vi "Meadowlark USB IO Example v1.1.VI"(0 "Set Voltage":dbl min=0.0 max=10.0 step=0.001 format="%.3f", 5 "error in (no error)":errorcluster) -> (14 "Readout \nVoltages":dbl[](array[numeric]) format="%.3f", 19 "error out":errorcluster)   [LabVIEW 2010]
doc: "This example selects channels and sets and reads voltages on a Meadowlark Optics D3040 Four-Cell controller. This VI can be opened and examined using LabVIEW (6.1 or newer) as a starting point for a user's custom development of a D3040 interface. Please note that the Sub-VI's used in this program require the file \"usbdrvd.dll\".\n\n(c) 2002-2003 Meadowlark Optics, Inc. All rights reserved."
panel:
  out "FW Version":dbl=2.0 min=0.0 max=10.0 step=0.001 format="%.2f"
  out "Update \nChannel":bool[](array[boolean])
  out "Located USB Devices":bool[](array[boolean])=[TRUE]
  in  "stop":bool
  in  "USB Device Number":i32=1 min=1 max=1
  in  "Channel":i32=1 min=1 max=4 step=1
  # "1"
  # "2"
  # "3"
  # "4"
  # "5"
  # "6"
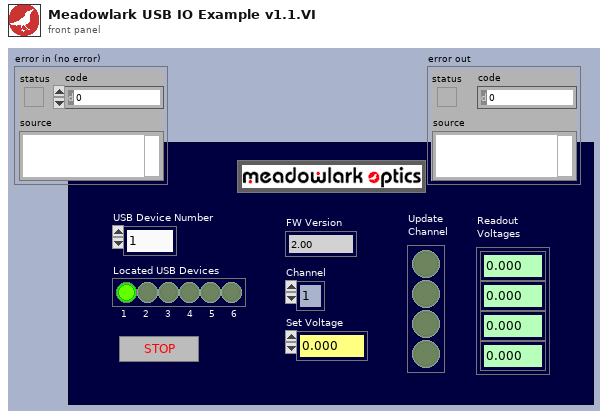
[diagram p1: front panel]
types:
  T1 = cluster{"Device Handle":u32, "Pipe 0 Handle":u32, "Pipe 1 Handle":u32}[]
  T2 = cluster{"Device Handle":u32, "Pipe 0 Handle":u32, "Pipe 1 Handle":u32}
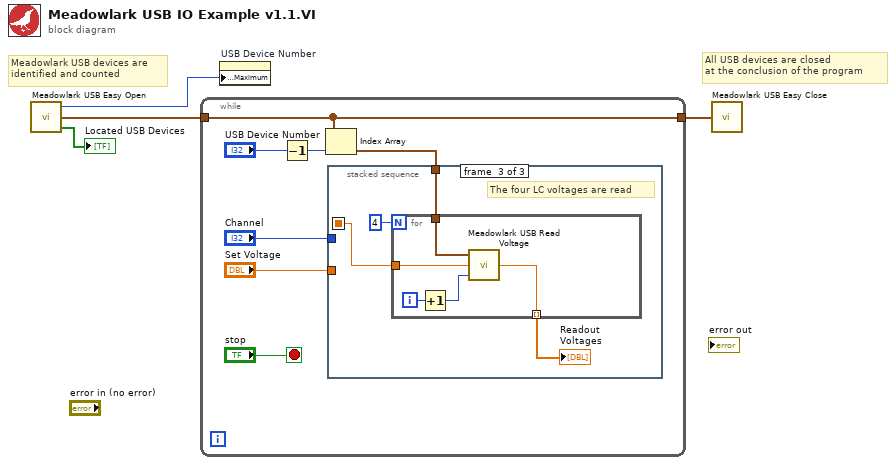
[diagram p0: block diagram]
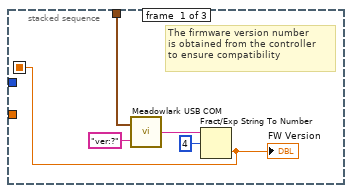
[diagram p2: hidden frame]
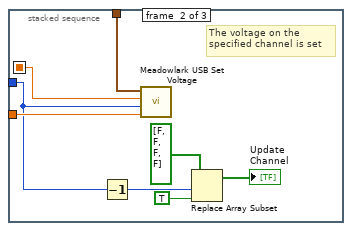
[diagram p3: hidden frame]
diagram:
  # "All USB devices are closed\nat the conclusion of the program"
  # "Meadowlark USB devices are\nidentified and counted"
  n1 = call "Meadowlark USB Easy Open.vi"() -> ("Device Opened Array"=→"Located USB Devices":bool[], "USB Device and Pipes Array"=w4:T1, "Device Count"=w2:u32)
  n2 = while {
    tunnel: w4 -> [w6]
    tunnel: [w6] -> w3
    stop <- "stop" stop-if-true
    n3 = Decrement(x="USB Device Number") -> (x-1=w8:i32)
    n4 = Index Array(array=w6, index=w8) -> (element=w5:T2)
    n5 = stacked-sequence {
      seq-local: [w12 _ _] -> [_ w17 w25]
      tunnel: "Set Voltage" -> [_ w24 _]
      tunnel: "Channel" -> [_ w20 _]
      tunnel: w5 -> [w16 w18 w26]
      frame #0 {
        # "The firmware version number\nis obtained from the controller\nto ensure compatibility"
        n6 = call "Meadowlark USB COM.vi"("WRITE IN String"="ver:?", "USB Open Device Cluster"=w16) -> ("READ OUT String"=w14:string)
        n7 = Fract/Exp String To Number(string=w14, offset=4) -> (number=w12:dbl)  [unwired: 2 in, 1 out]
        "FW Version" <- w12
      }
      frame #1 {
        # "The voltage on the\nspecified channel is set"
        n8 = Decrement(x=w20) -> (x-1=w23:i32)
        n9 = call "Meadowlark USB Set Voltage.VI"("LC Voltage"=w24, "LC Channel"=w20, "FW Version"=w17, "USB Open Device Cluster"=w18) -> ()  [unwired: 1 out]
        n10 = Replace Array Subset(array=bool[] [FALSE, FALSE, FALSE, FALSE], new element=TRUE ("new element/subarray"), index=w23) -> (→"Update \nChannel":bool[])
      }
      frame #2 {
        # "The four LC voltages are read"
        n11 = for {
          N: 4 -> [_]
          tunnel: [w32] -> w27 mode=indexing
          tunnel: w26 -> [w31]
          tunnel: w25 -> [w29]
          i -> [w33]
          n12 = Increment(x=w33) -> (x+1=w30:i32)
          n13 = call "Meadowlark USB Read Voltage.VI"("LC Channel"=w30, "FW Version"=w29, "USB Open Device Cluster"=w31) -> ("Readout \nVoltage"=w32:dbl)
        }
        "Readout \nVoltages" <- w27
      }
    }
  }
  n14 = property on="USB Device Number" class="DigNum (strict)"("Data Entry Limits:Maximum"=w2) -> ()  [unwired: 2 in, 2 out]
  n15 = call "Meadowlark USB Easy Close.vi"("USB Device and Pipes Array"=w3) -> ()
